vi "Modbus Speed Test.vi"() -> ()   [LabVIEW 2015]
doc: "Tests client-server connection and measures transaction time."
uses:
  <vilib>/Utility/error.llb/DialogType.ctl
  PL Modbus Client.lvclass
panel:
  in  "interface":enum32{"serial", "TCP"}(tab)
  in  "serial settings":T1={"port"="", "protocol"=enum."RTU", "address"=1, "baud rate"=9600, "data bits"=8, "parity"=enum."Even", "stop bits"=10, "flow control"=0} {"flow control" items=["None", "XON/XOFF", "RTS/CTS", "XON/XOFF & RTS/CTS", "DTR/DSR", "XON/XOFF & DTR/DSR"]; "stop bits" items=["1.0"=10, "1.5"=15, "2.0"=20]}
  in  "TCP settings":T2={"ip address"="192.168.1.1", "port"=502, "station address"=255}
  out "error":string
  in  "number of items":u16=8
  in  "data address":u16
  in  "method":u16(ring) items=["read coils", "read discrete inputs", "read holding registers", "read input registers"]
  in  "timeout, ms":u32=300
  in  "stop":bool
  out "transaction time, ms":u32
  out "transactions":i32
  out "errors":u32
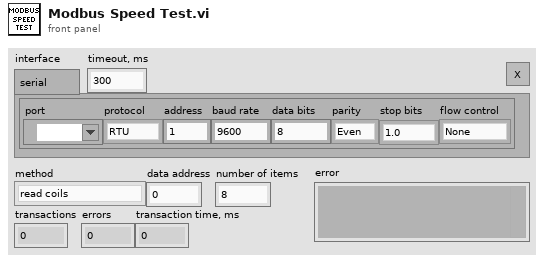
[diagram p1: front panel]
types:
  T1 = cluster{"port":refnum<visa-resource-name>, "protocol":enum16{"RTU", "ASCII"}, "address":u8, "baud rate":u32, "data bits":u16, "parity":enum16{"None", "Odd", "Even", "Mark", "Space"}, "stop bits":u16, "flow control":u16}
  T2 = cluster{"ip address":string, "port":u16, "station address":u8}
  T3 = typedef "DialogType.ctl" = u16
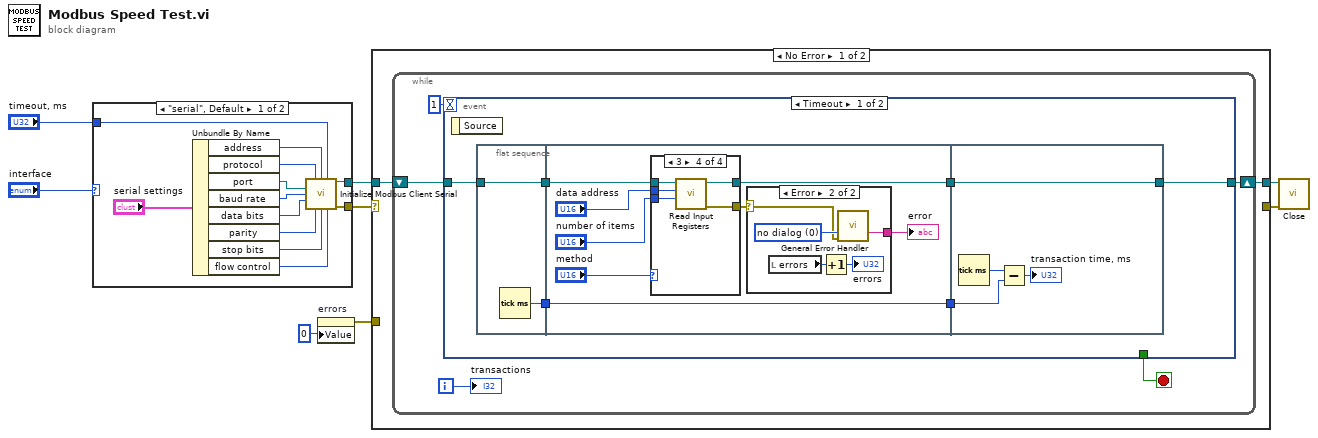
[diagram p0: block diagram]
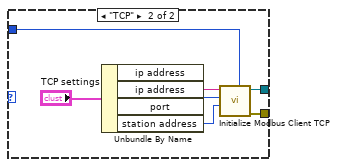
[diagram p2: hidden frame]
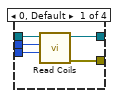
[diagram p3: hidden frame]
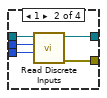
[diagram p4: hidden frame]
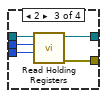
[diagram p5: hidden frame]
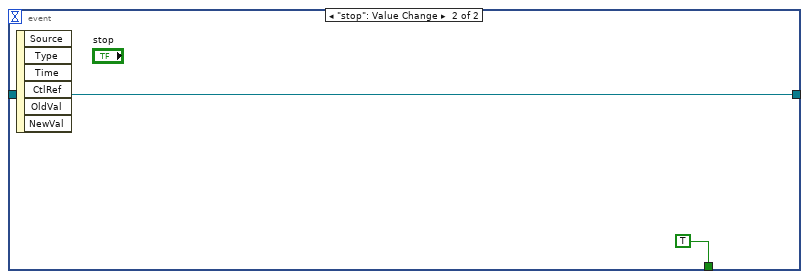
[diagram p7: hidden frame]
diagram:
  n1 = case shown="\"serial\", Default" "interface" {
    tunnel: [w20 w25] -> w4
    tunnel: [w19 w24] -> w3
    tunnel: "timeout, ms" -> [w11 w21]
    frame "serial", Default {
      n2 = Unbundle By Name("serial settings") -> ("address"=w10:u8, "protocol"=w9:enum16{"RTU", "ASCII"}, "port"=w18:refnum<visa-resource-name>, "baud rate"=w13:u32, "data bits"=w14:u16, "parity"=w15:enum16{"None", "Odd", "Even", "Mark", "Space"}, "stop bits"=w16:u16, "flow control"=w17:u16)
      n3 = call "Initialize Modbus Client Serial.vi"("protocol (RTU)"=w9, "station address (1)"=w10, "timeout, ms (300)"=w11, "port"=w18, "baud rate (9600)"=w13, "data bits (8)"=w14, "parity (even)"=w15, "stop bits (1.0)"=w16, "flow control (none)"=w17) -> ("MODBUS out"=w20:refnum<class "PL Modbus Client.lvclass">, "error out"=w19:errorcluster)  [unwired: 5 in]
    }
    frame "TCP" {
      n4 = Unbundle By Name("TCP settings") -> ("ip address"=w27:string, "port"=w26:u16, "station address"=w22:u8)  [unwired: 1 out]
      n5 = call "Initialize Modbus Client TCP.vi"("timeout, ms (300)"=w21, "station address (255)"=w22, "port (502)"=w26, "ip address"=w27) -> ("error out"=w24:errorcluster, "MODBUS out"=w25:refnum<class "PL Modbus Client.lvclass">)  [unwired: 6 in]
    }
  }
  n6 = property on="errors" class="DigNum (strict)"("Value"=u32 0 ("errors")) -> (error out=w7:errorcluster)  [unwired: 2 in, 1 out]
  n7 = case shown="No Error" w3 {
    selector: w3 -> [_ w82]
    tunnel: [w28 w83] -> w8
    tunnel: w4 -> [w29 w83]
    tunnel: w7 -> [_ _]
    tunnel: [_ w82] -> w1
    frame No Error {
      n8 = while {
        shift-right: [w33] -> w28
        shift-left: w29 -> [w34]
        i -> [w31]
        stop <- w32 stop-if-true
        n9 = event shown="[0] Timeout" {
          selector: _ -> [_ _]
          dyn-events: _ -> [_ _]
          timeout: 1 -> [_ _]
          tunnel: w34 -> [w40 w80]
          tunnel: [w39 w80] -> w33
          tunnel: [_ TRUE] -> w32
          event Timeout {
            n10 = event-data() -> ()  [unwired: 1 in, 1 out]
            n11 = flat-sequence {
              tunnel: w40 -> [w42]
              tunnel: [w42] -> w38
              tunnel: [w41] -> w37
              tunnel: w38 -> [w48]
              tunnel: w37 -> [w50]
              tunnel: [w47] -> w36
              tunnel: [w50] -> w35
              tunnel: [w79] -> w39
              tunnel: w36 -> [w79]
              tunnel: w35 -> [w77]
              frame #0 {
                n12 = Tick Count (ms)() -> (millisecond timer value=w41:u32)
              }
              frame #1 {
                n13 = case shown="3" "method" {
                  tunnel: w48 -> [w55 w60 w65 w70]
                  tunnel: [w54 w59 w64 w69] -> w47
                  tunnel: "data address" -> [w53 w58 w63 w68]
                  tunnel: "number of items" -> [w52 w57 w62 w67]
                  tunnel: [w51 w56 w61 w66] -> w44
                  frame 0, Default {
                    n14 = call "Read Coils.vi"("number of coils"=w52, "address"=w53, "MODBUS in"=w55) -> ("error out"=w51:errorcluster, "MODBUS out"=w54:refnum<class "PL Modbus Client.lvclass">)  [unwired: 6 in, 1 out]
                  }
                  frame 1 {
                    n15 = call "Read Discrete Inputs.vi"("number of discrete inputs"=w57, "address"=w58, "MODBUS in"=w60) -> ("error out"=w56:errorcluster, "MODBUS out"=w59:refnum<class "PL Modbus Client.lvclass">)  [unwired: 6 in, 1 out]
                  }
                  frame 2 {
                    n16 = call "Read Holding Registers.vi"("number of holding registers"=w62, "address"=w63, "MODBUS in"=w65) -> ("error out"=w61:errorcluster, "MODBUS out"=w64:refnum<class "PL Modbus Client.lvclass">)  [unwired: 6 in, 1 out]
                  }
                  frame 3 {
                    n17 = call "Read Input Registers.vi"("number of input registers"=w67, "address"=w68, "MODBUS in"=w70) -> ("error out"=w66:errorcluster, "MODBUS out"=w69:refnum<class "PL Modbus Client.lvclass">)  [unwired: 6 in, 1 out]
                  }
                }
                n18 = case shown="Error" w44 {
                  selector: w44 -> [_ w72]
                  tunnel: [_ w71] -> w43
                  frame No Error {
                  }
                  frame Error {
                    w73 = T3 0 items=["no dialog", "OK message", "continue or stop message", "OK message + warnings", "continue/stop + warnings"] ("type of dialog (OK msg:1)")
                    n19 = local read "errors"() -> (w75:u32)
                    n20 = Increment(x=w75) -> (x+1=→"errors":u32)
                    n21 = call <vilib>:"General Error Handler.vi"("type of dialog (OK msg:1)"=w73, "error in (no error)"=w72) -> ("message"=w71:string)  [unwired: 9 in, 4 out]
                  }
                }
                "error" <- w43
              }
              frame #2 {
                n22 = Tick Count (ms)() -> (millisecond timer value=w78:u32)
                n23 = Subtract(x=w78, y=w77) -> (x-y=→"transaction time, ms":u32)
              }
            }
          }
          event "stop": Value Change {
            n24 = event-data() -> ()  [unwired: 1 in, 6 out]
          }
        }
        "transactions" <- w31
      }
    }
    frame Error {
    }
  }
  n25 = call-dynamic "Close.vi"("error in (no error)"=w1, "MODBUS in"=w8) -> ()  [unwired: 9 in, 1 out]
